vi "Alignment (2).vi"() -> ()   [LabVIEW 2010]
uses:
  <vilib>/Utility/inputDevices.llb/closeKeyboard.vi
  <vilib>/Utility/inputDevices.llb/keyboardAcquire.vi
panel:
  out "Q":bool
  out "Further":bool
  out "Nearer":bool
  out "End":bool=TRUE
  out "Right":bool
  out "Up":bool
  out "Left":bool
  out "Down":bool
  in  "Motor GPIB":u8=6 max=32 step=1 format="%#.0f"
  out "keys pressed":T1(array[ring])
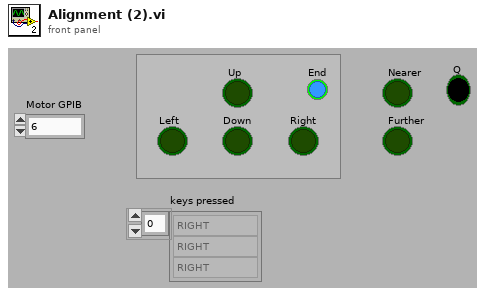
[diagram p1: front panel]
types:
  T1 = enum16{"0", "1", "2", "3", "4", "5", "6", "7", "8", "9", "A", "B", "C", "D", "E", "F", "G", "H", "I", "J", "K", "L", "M", "N", "O", "P", "Q", "R", "S", "T", "U", "V", "W", "X", "Y", "Z", "F1", "F2", "F3", "F4", "F5", "F6", "F7", "F8", "F9", "F10", "F11", "F12", "F13", "F14", "F15", "ADD", "BACK", "BACKSLASH", "CAPITAL", "COMMA", "DECIMAL", "DELETE", "DIVIDE", "DOWN", "END", "EQUALS", "ESCAPE", "GRAVE (`)", "HOME", "INSERT", "LBRACKET", "LCONTROL", "LEFT", "L ALT", "LSHIFT", "LWIN", "MINUS", "MULTIPLY", "NEXT", "NUMLOCK", "NUMPAD_0", "NUMPAD_1", "NUMPAD_2", "NUMPAD_3", "NUMPAD_4", "NUMPAD_5", "NUMPAD_6", "NUMPAD_7", "NUMPAD_8", "NUMPAD_9", "PAUSE", "PERIOD", "PRIOR (PG UP)", "RBRACKET", "RCONTROL", "RETURN", "RIGHT", "R ALT", "RSHIFT", "RWIN", "SCROLL", "SEMICOLON", "SLASH", "SPACE", "SUBTRACT", "TAB", "UP", "ENTER (num pad)", "' (quote)"}[]
  T2 = enum16{"0", "1", "2", "3", "4", "5", "6", "7", "8", "9", "A", "B", "C", "D", "E", "F", "G", "H", "I", "J", "K", "L", "M", "N", "O", "P", "Q", "R", "S", "T", "U", "V", "W", "X", "Y", "Z", "F1", "F2", "F3", "F4", "F5", "F6", "F7", "F8", "F9", "F10", "F11", "F12", "F13", "F14", "F15", "ADD", "BACK", "BACKSLASH", "CAPITAL", "COMMA", "DECIMAL", "DELETE", "DIVIDE", "DOWN", "END", "EQUALS", "ESCAPE", "GRAVE (`)", "HOME", "INSERT", "LBRACKET", "LCONTROL", "LEFT", "L ALT", "LSHIFT", "LWIN", "MINUS", "MULTIPLY", "NEXT", "NUMLOCK", "NUMPAD_0", "NUMPAD_1", "NUMPAD_2", "NUMPAD_3", "NUMPAD_4", "NUMPAD_5", "NUMPAD_6", "NUMPAD_7", "NUMPAD_8", "NUMPAD_9", "PAUSE", "PERIOD", "PRIOR (PG UP)", "RBRACKET", "RCONTROL", "RETURN", "RIGHT", "R ALT", "RSHIFT", "RWIN", "SCROLL", "SEMICOLON", "SLASH", "SPACE", "SUBTRACT", "TAB", "UP", "ENTER (num pad)", "' (quote)"}
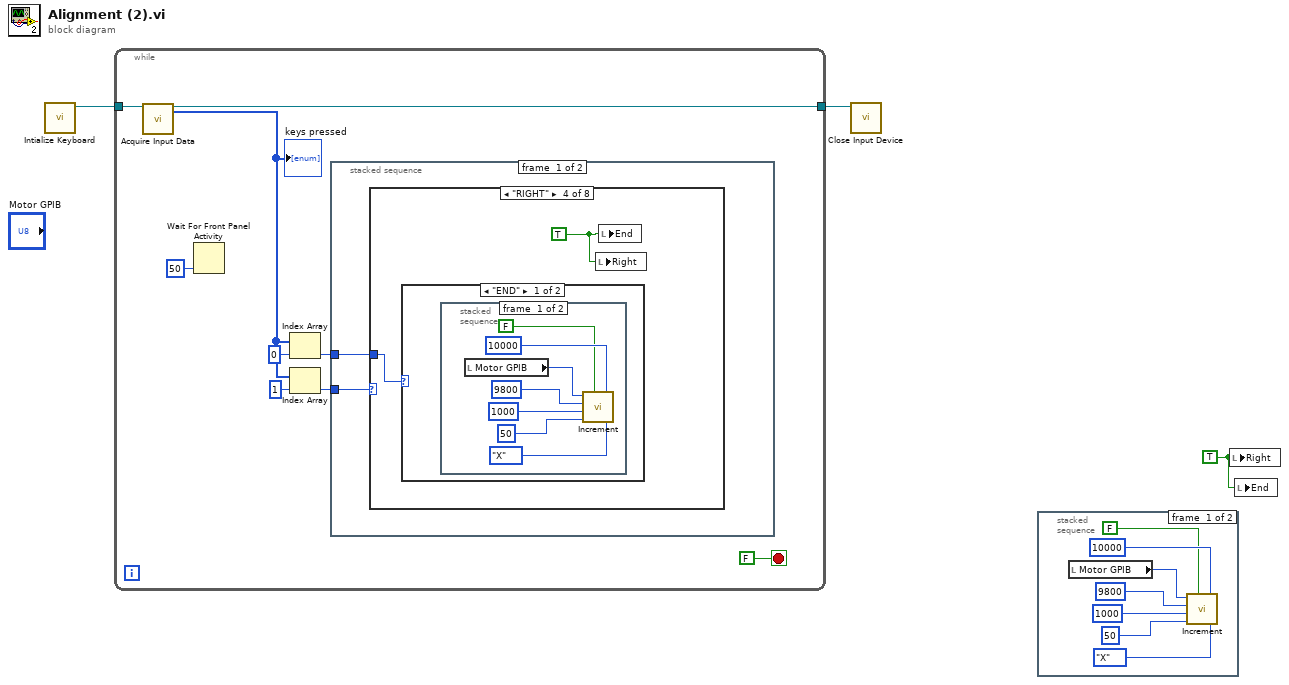
[diagram p0: block diagram]
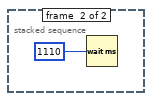
[diagram p2: hidden frame]
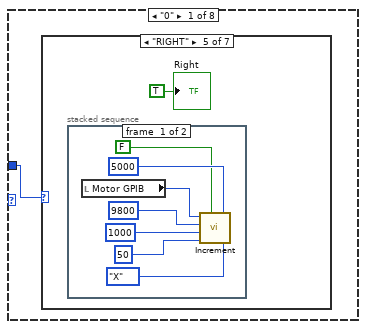
[diagram p3: hidden frame]
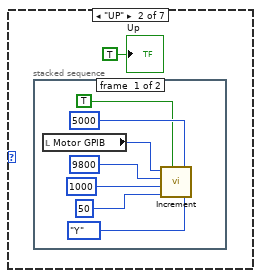
[diagram p5: hidden frame]
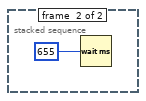
[diagram p6: hidden frame]
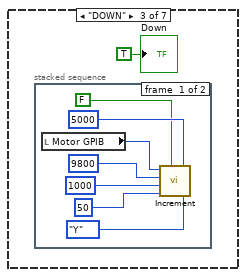
[diagram p7: hidden frame]
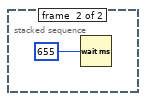
[diagram p8: hidden frame]
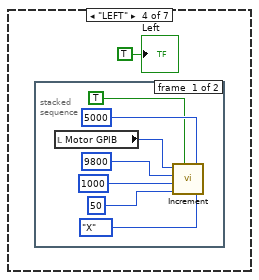
[diagram p9: hidden frame]
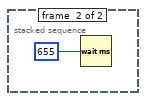
[diagram p10: hidden frame]
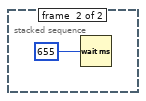
[diagram p11: hidden frame]
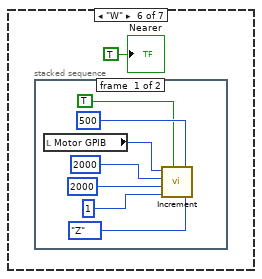
[diagram p12: hidden frame]
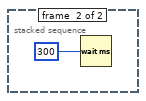
[diagram p13: hidden frame]
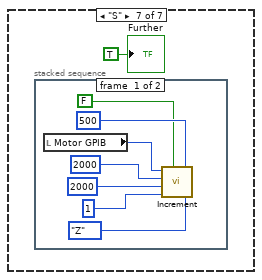
[diagram p14: hidden frame]
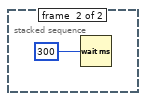
[diagram p15: hidden frame]
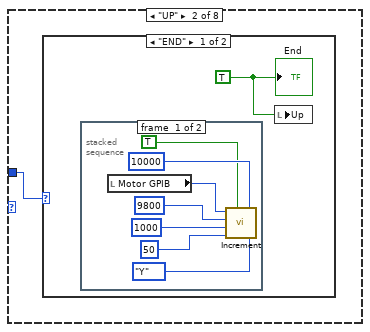
[diagram p16: hidden frame]
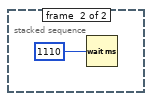
[diagram p17: hidden frame]
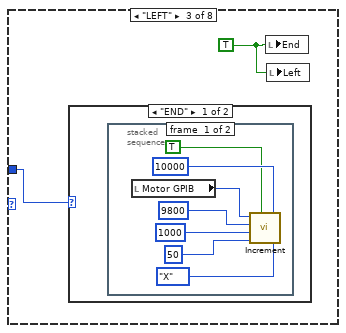
[diagram p19: hidden frame]
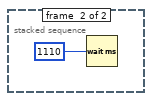
[diagram p20: hidden frame]
diagram:
  w1 = TRUE ("Ctrl")
  n1 = call <vilib>:"Intialize Keyboard.vi"() -> ("device ID"=w2:refnum<k1>)  [unwired: 10 in, 1 out]
  n2 = while {
    tunnel: w2 -> [w12]
    tunnel: [w11] -> w3
    stop <- FALSE stop-if-true
    n3 = call-poly <vilib>:"Acquire Input Data.vi"("device ID"=w12) -> ("device ID"=w11:refnum<k1>, "keys pressed"=w9:T1)  [unwired: 16 in, 1 out]
    "keys pressed" <- w9
    n4 = Wait For Front Panel Activity(1:50 ("timeout ms (-1 never timeout)")) -> ()  [unwired: 2 in, 1 out]
    n5 = Index Array(array=w9, index=0) -> (element=w5:T2)
    n6 = Index Array(array=w9, index=1) -> (element=w6:T2)
    n7 = stacked-sequence {
      tunnel: w6 -> [w14 _]
      tunnel: w5 -> [w13 _]
      frame #0 {
        n8 = case shown="\"RIGHT\"" w14 {
          tunnel: w13 -> [w15 w70 w80 w91 w100 w110 w120 _]
          frame "0" {
            n9 = case shown="\"RIGHT\"" w15 {
              frame "0", Default {
              }
              frame "UP" {
                n10 = stacked-sequence {
                  frame #0 {
                    n11 = local read "Motor GPIB"() -> (w23:u8)
                    n12 = call "Increment.vi"("GPIB_Addr"=w23, "F Speed"=u16 9800, "L Speed"=u16 1000, "Rate"=u16 50, "CCW 3"=TRUE, "Distance"=u32 5000, "Axis"=enum16{"X", "Y", "Z", "U", "V", "W"}."Y") -> ()
                  }
                  frame #1 {
                    n13 = Wait (ms)(milliseconds to wait=655 ("timeout ms (-1 never timeout)")) -> ()  [unwired: 1 out]
                  }
                }
                "Up" <- TRUE ("Up")
              }
              frame "DOWN" {
                n14 = stacked-sequence {
                  frame #0 {
                    n15 = local read "Motor GPIB"() -> (w32:u8)
                    n16 = call "Increment.vi"("GPIB_Addr"=w32, "F Speed"=u16 9800, "L Speed"=u16 1000, "Rate"=u16 50, "CCW 3"=FALSE, "Distance"=u32 5000, "Axis"=enum16{"X", "Y", "Z", "U", "V", "W"}."Y") -> ()
                  }
                  frame #1 {
                    n17 = Wait (ms)(milliseconds to wait=655 ("timeout ms (-1 never timeout)")) -> ()  [unwired: 1 out]
                  }
                }
                "Down" <- TRUE ("Down")
              }
              frame "LEFT" {
                n18 = stacked-sequence {
                  frame #0 {
                    n19 = local read "Motor GPIB"() -> (w41:u8)
                    n20 = call "Increment.vi"("GPIB_Addr"=w41, "F Speed"=u16 9800, "L Speed"=u16 1000, "Rate"=u16 50, "CCW 3"=TRUE, "Distance"=u32 5000, "Axis"=enum16{"X", "Y", "Z", "U", "V", "W"}."X") -> ()
                  }
                  frame #1 {
                    n21 = Wait (ms)(milliseconds to wait=655 ("timeout ms (-1 never timeout)")) -> ()  [unwired: 1 out]
                  }
                }
                "Left" <- TRUE ("Left")
              }
              frame "RIGHT" {
                n22 = stacked-sequence {
                  frame #0 {
                    n23 = local read "Motor GPIB"() -> (w50:u8)
                    n24 = call "Increment.vi"("GPIB_Addr"=w50, "F Speed"=u16 9800, "L Speed"=u16 1000, "Rate"=u16 50, "CCW 3"=FALSE, "Distance"=u32 5000, "Axis"=enum16{"X", "Y", "Z", "U", "V", "W"}."X") -> ()
                  }
                  frame #1 {
                    n25 = Wait (ms)(milliseconds to wait=655 ("timeout ms (-1 never timeout)")) -> ()  [unwired: 1 out]
                  }
                }
                "Right" <- TRUE ("Right")
              }
              frame "W" {
                n26 = stacked-sequence {
                  frame #0 {
                    n27 = local read "Motor GPIB"() -> (w59:u8)
                    n28 = call "Increment.vi"("GPIB_Addr"=w59, "F Speed"=u16 2000, "L Speed"=u16 2000, "Rate"=u16 1, "CCW 3"=TRUE, "Distance"=u32 500, "Axis"=enum16{"X", "Y", "Z", "U", "V", "W"}."Z") -> ()
                  }
                  frame #1 {
                    n29 = Wait (ms)(milliseconds to wait=300 ("timeout ms (-1 never timeout)")) -> ()  [unwired: 1 out]
                  }
                }
                "Nearer" <- TRUE ("Up")
              }
              frame "S" {
                n30 = stacked-sequence {
                  frame #0 {
                    n31 = local read "Motor GPIB"() -> (w68:u8)
                    n32 = call "Increment.vi"("GPIB_Addr"=w68, "F Speed"=u16 2000, "L Speed"=u16 2000, "Rate"=u16 1, "CCW 3"=FALSE, "Distance"=u32 500, "Axis"=enum16{"X", "Y", "Z", "U", "V", "W"}."Z") -> ()
                  }
                  frame #1 {
                    n33 = Wait (ms)(milliseconds to wait=300 ("timeout ms (-1 never timeout)")) -> ()  [unwired: 1 out]
                  }
                }
                "Further" <- TRUE ("Up")
              }
            }
          }
          frame "UP" {
            n34 = case shown="\"END\"" w70 {
              frame "END" {
                w71 = TRUE ("RCtrl")
                n35 = stacked-sequence {
                  frame #0 {
                    n36 = local read "Motor GPIB"() -> (w78:u8)
                    n37 = call "Increment.vi"("GPIB_Addr"=w78, "F Speed"=u16 9800, "L Speed"=u16 1000, "Rate"=u16 50, "CCW 3"=TRUE, "Distance"=u32 10000, "Axis"=enum16{"X", "Y", "Z", "U", "V", "W"}."Y") -> ()
                  }
                  frame #1 {
                    n38 = Wait (ms)(milliseconds to wait=1110 ("timeout ms (-1 never timeout)")) -> ()  [unwired: 1 out]
                  }
                }
                n39 = local write "Up"(w71) -> ()
                "End" <- w71
              }
              frame "2", Default {
              }
            }
          }
          frame "LEFT" {
            w81 = TRUE ("CCW 3")
            n40 = case shown="\"END\"" w80 {
              frame "END" {
                n41 = stacked-sequence {
                  frame #0 {
                    n42 = local read "Motor GPIB"() -> (w88:u8)
                    n43 = call "Increment.vi"("GPIB_Addr"=w88, "F Speed"=u16 9800, "L Speed"=u16 1000, "Rate"=u16 50, "CCW 3"=TRUE, "Distance"=u32 10000, "Axis"=enum16{"X", "Y", "Z", "U", "V", "W"}."X") -> ()
                  }
                  frame #1 {
                    n44 = Wait (ms)(milliseconds to wait=1110 ("timeout ms (-1 never timeout)")) -> ()  [unwired: 1 out]
                  }
                }
              }
              frame "2", Default {
              }
            }
            n45 = local write "End"(w81) -> ()
            n46 = local write "Left"(w81) -> ()
          }
          frame "RIGHT" {
            w90 = TRUE ("CCW 3")
            n47 = case shown="\"END\"" w91 {
              frame "END" {
                n48 = stacked-sequence {
                  frame #0 {
                    n49 = local read "Motor GPIB"() -> (w98:u8)
                    n50 = call "Increment.vi"("GPIB_Addr"=w98, "F Speed"=u16 9800, "L Speed"=u16 1000, "Rate"=u16 50, "CCW 3"=FALSE, "Distance"=u32 10000, "Axis"=enum16{"X", "Y", "Z", "U", "V", "W"}."X") -> ()
                  }
                  frame #1 {
                    n51 = Wait (ms)(milliseconds to wait=1110 ("timeout ms (-1 never timeout)")) -> ()  [unwired: 1 out]
                  }
                }
              }
              frame "2", Default {
              }
            }
            n52 = local write "Right"(w90) -> ()
            n53 = local write "End"(w90) -> ()
          }
          frame "END" {
            n54 = case shown="\"DOWN\"" w100 {
              frame "0", Default {
              }
              frame "DOWN" {
                w101 = TRUE ("Ctrl")
                n55 = stacked-sequence {
                  frame #0 {
                    n56 = local read "Motor GPIB"() -> (w108:u8)
                    n57 = call "Increment.vi"("GPIB_Addr"=w108, "F Speed"=u16 9800, "L Speed"=u16 1000, "Rate"=u16 50, "CCW 3"=FALSE, "Distance"=u32 10000, "Axis"=enum16{"X", "Y", "Z", "U", "V", "W"}."Y") -> ()
                  }
                  frame #1 {
                    n58 = Wait (ms)(milliseconds to wait=1110 ("timeout ms (-1 never timeout)")) -> ()  [unwired: 1 out]
                  }
                }
                n59 = local write "End"(w101) -> ()
                n60 = local write "Down"(w101) -> ()
              }
            }
          }
          frame "W" {
            n61 = case shown="\"Q\"" w110 {
              frame "7", Default {
              }
              frame "Q" {
                w111 = TRUE ("Up")
                n62 = stacked-sequence {
                  frame #0 {
                    n63 = local read "Motor GPIB"() -> (w118:u8)
                    n64 = call "Increment.vi"("GPIB_Addr"=w118, "F Speed"=u16 9999, "L Speed"=u16 9999, "Rate"=u16 1, "CCW 3"=FALSE, "Distance"=u32 3000, "Axis"=enum16{"X", "Y", "Z", "U", "V", "W"}."Z") -> ()
                  }
                  frame #1 {
                    n65 = Wait (ms)(milliseconds to wait=300 ("timeout ms (-1 never timeout)")) -> ()  [unwired: 1 out]
                  }
                }
                n66 = local write "Nearer"(w111) -> ()
                "Q" <- w111
              }
            }
          }
          frame "S" {
            n67 = case shown="\"Q\"" w120 {
              frame "7", Default {
              }
              frame "Q" {
                w121 = TRUE ("Up")
                n68 = stacked-sequence {
                  frame #0 {
                    n69 = local read "Motor GPIB"() -> (w128:u8)
                    n70 = call "Increment.vi"("GPIB_Addr"=w128, "F Speed"=u16 9999, "L Speed"=u16 9999, "Rate"=u16 1, "CCW 3"=TRUE, "Distance"=u32 3000, "Axis"=enum16{"X", "Y", "Z", "U", "V", "W"}."Z") -> ()
                  }
                  frame #1 {
                    n71 = Wait (ms)(milliseconds to wait=300 ("timeout ms (-1 never timeout)")) -> ()  [unwired: 1 out]
                  }
                }
                n72 = local write "Further"(w121) -> ()
                n73 = local write "Q"(w121) -> ()
              }
            }
          }
          frame "2", Default {
          }
        }
      }
      frame #1 {
        w130 = FALSE ("Up")
        n74 = local write "Up"(w130) -> ()
        n75 = local write "Down"(w130) -> ()
        n76 = local write "Left"(w130) -> ()
        n77 = local write "Right"(w130) -> ()
        n78 = local write "End"(w130) -> ()
        n79 = local write "Further"(w130) -> ()
        n80 = local write "Nearer"(w130) -> ()
        n81 = local write "Q"(w130) -> ()
      }
    }
  }
  n82 = call-poly <vilib>:"Close Input Device.vi"("device ID"=w3) -> ()  [unwired: 9 in, 1 out]
  n83 = stacked-sequence {
    frame #0 {
      n84 = local read "Motor GPIB"() -> (w137:u8)
      n85 = call "Increment.vi"("GPIB_Addr"=w137, "F Speed"=u16 9800, "L Speed"=u16 1000, "Rate"=u16 50, "CCW 3"=FALSE, "Distance"=u32 10000, "Axis"=enum16{"X", "Y", "Z", "U", "V", "W"}."X") -> ()
    }
    frame #1 {
      n86 = Wait (ms)(milliseconds to wait=1110 ("timeout ms (-1 never timeout)")) -> ()  [unwired: 1 out]
    }
  }
  n87 = local write "Right"(w1) -> ()
  n88 = local write "End"(w1) -> ()
